vi "DisposeCore.vi"(8 "error in (no error)":errorcluster, 11 "Wall":refnum<class "Wall.lvclass">) -> (0 "error out":errorcluster, 3 "Wall":refnum<class "Wall.lvclass">)   [LabVIEW 2020, in "Wall.lvclass"]
uses:
  Wall.lvclass
  Private/TypeDef/privateDataDVR.ctl
  Private/TypeDef/privateData.ctl
  Wall.lvclass/Wall.ctl
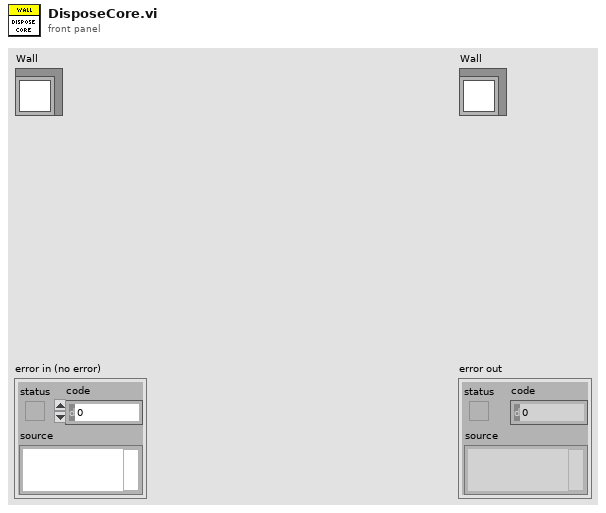
[diagram p1: front panel]
types:
  T1 = typedef "Wall.lvclass/privateDataDVR.ctl" = refnum<data-value>
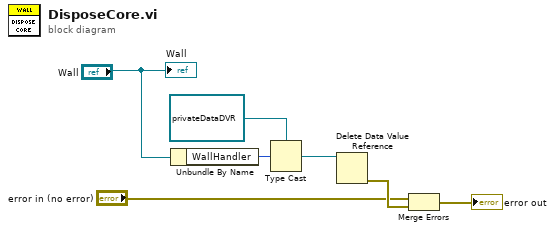
[diagram p0: block diagram]
diagram:
  n1 = Unbundle By Name("Wall") -> ("WallHandler"=w6:u32)
  n2 = Type Cast(type=T1 refnum ("privateDataDVR"), x=w6) -> (*(type *) &x=w7:T1)
  n3 = Delete Data Value Reference(data value reference=w7) -> (error out=w5:errorcluster)  [unwired: 1 in, 1 out]
  n4 = Merge Errors("error in (no error)", w5) -> (→"error out":errorcluster)
  "Wall" <- "Wall"
